vi "Start.vi"(8 "error in (no error)":errorcluster caption="错误输入（无错误）", 11 "Primary Productivity 输入":refnum<class "Primary Productivity.lvclass">) -> (0 "error out":errorcluster caption="错误输出", 3 "Primary Productivity 输出":refnum<class "Primary Productivity.lvclass">)   [LabVIEW 2016, in "Primary Productivity.lvclass"]
uses:
  Primary Productivity.lvclass
  <vilib>/Instr/_visa.llb/VISA Flush IO Buffer Mask.ctl
  Primary Productivity.lvclass/Primary Productivity.ctl
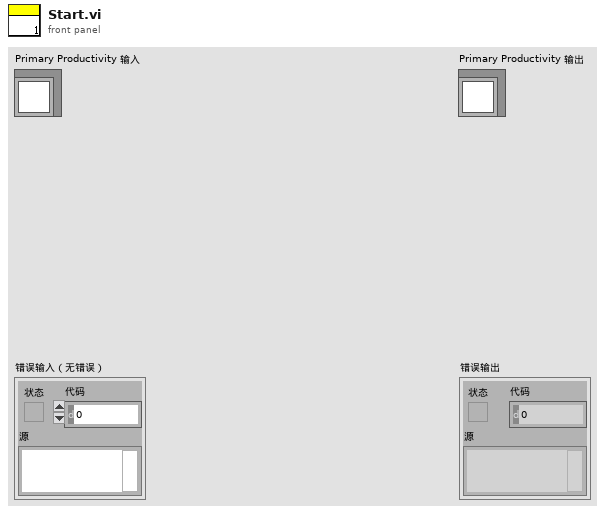
[diagram p1: front panel]
types:
  T1 = typedef "VISA Flush IO Buffer Mask.ctl" = u16
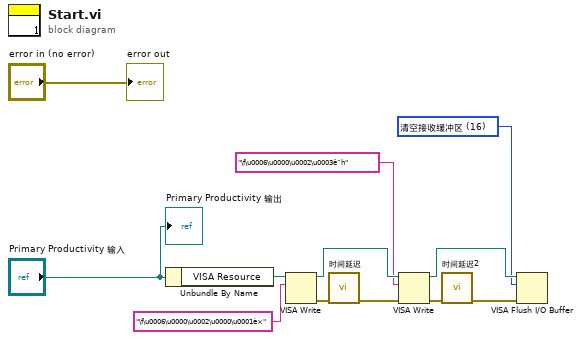
[diagram p0: block diagram]
diagram:
  w1 = T1 16 items=["清空接收缓冲区"=16, "向设备写入传输缓冲区"=32, "清空接收缓冲区（无I/O）"=64, "清空传输缓冲区"=128] ("Mask")
  n1 = Unbundle By Name("Primary Productivity 输入") -> ("VISA Resource"=w5:refnum<visa-resource-name>)
  n2 = VISA Write(VISA resource name=w5, write buffer="\f\u0006\u0000\u0002\u0000\u0001è×" ("写入缓冲区")) -> (VISA resource name out=w7:refnum<visa-resource-name>, error out=w9:errorcluster)  [unwired: 1 in, 1 out]
  n3 = call "时间延迟"("error in (no error)"=w9) -> ("error out"=w8:errorcluster)  [unwired: 10 in]
  n4 = VISA Write(VISA resource name=w7, write buffer="\f\u0006\u0000\u0002\u0003ê¨h" ("写入缓冲区"), error in (no error)=w8) -> (VISA resource name out=w3:refnum<visa-resource-name>, error out=w4:errorcluster)  [unwired: 1 out]
  n5 = call "时间延迟2"("error in (no error)"=w4) -> ("error out"=w2:errorcluster)  [unwired: 10 in]
  n6 = VISA Flush I/O Buffer(VISA resource name=w3, mask (16)=w1, error in (no error)=w2) -> ()  [unwired: 2 out]
  "error out" <- "error in (no error)"
  "Primary Productivity 输出" <- "Primary Productivity 输入"
